vi "h.vi"(9 "Interval Units":enum16{"Points", "Data"}(ring), 10 "Interval (h)":dbl, 11 "X-array":dbl[](array[numeric])) -> ()   [LabVIEW 2016, in "xy_utilities.lvlib"]
doc: "Calculate <b>h</b> in appropriate units."
uses:
  xy_utilities.lvlib
panel:
  out "h":i32
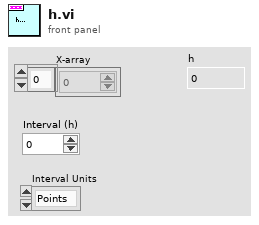
[diagram p1: front panel]
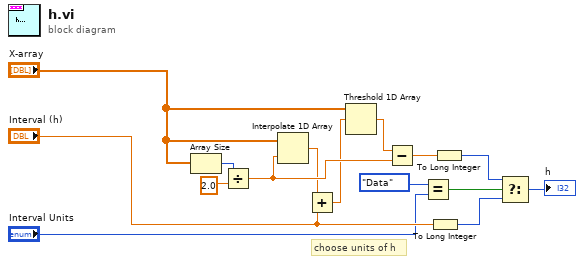
[diagram p0: block diagram]
diagram:
  # "choose units of h"
  n1 = Array Size(array="X-array") -> (size(s)=w8:i32)
  n2 = Divide(x=w8, y=2.0) -> (x/y=w10:dbl)
  n3 = Interpolate 1D Array(1:w10, 2:"X-array") -> (0:w9:dbl)
  n4 = Add(x=w9, y="Interval (h)") -> (x+y=w5:dbl)
  n5 = Threshold 1D Array(2:w5, 3:"X-array") -> (0:w4:dbl)  [unwired: 1 in]
  n6 = Subtract(x=w4, y=w10) -> (x-y=w13:dbl)
  n7 = Equal?(x=enum16{"Points", "Data"}."Data" ("Interval Units"), y="Interval Units") -> (x = y?=w7:bool)
  n8 = To Long Integer(number="Interval (h)") -> (32bit integer=w15:i32)
  n9 = To Long Integer(number=w13) -> (32bit integer=w14:i32)
  n10 = Select(t=w14, s=w7, f=w15) -> (s? t:f=→"h":i32)
